vi "Set Input Volume.vi"(7 "Volume Mode (dB)":T1, 8 "error in (no error)":errorcluster, 9 "Volume":dbl, 10 "Input Name":string, 11 "OBS in":refnum<class "OBS.lvclass">) -> (0 "error out":errorcluster, 3 "OBS out":refnum<class "OBS.lvclass">)   [LabVIEW 2020, in "obs-websocket.lvlib" / "OBS.lvclass"]
uses:
  OBS.lvclass
  OBS.lvclass/OBS.ctl
  SetInputVolume/SetInputVolume.lvclass
  Volume Mode.ctl
  obs-websocket.lvlib
  C:/dev/lv20CE/lv-obs-websocket/obs-websocket-lv/Request/Request.lvclass
  C:/dev/lv20CE/lv-obs-websocket/obs-websocket-lv/Client Message/Client Message.lvclass
  C:/dev/lv20CE/lv-obs-websocket/obs-websocket-lv/Message/Message.lvclass
  C:/dev/lv20CE/lv-obs-websocket/obs-websocket-lv/SetInputVolume/SetInputVolume.lvclass
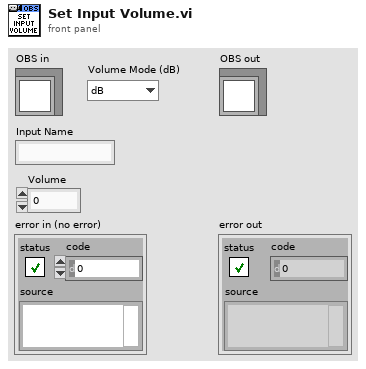
[diagram p1: front panel]
types:
  T1 = typedef "obs-websocket.lvlib/Volume Mode.ctl" = enum16{"dB", "Mul"}
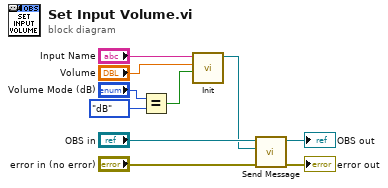
[diagram p0: block diagram]
diagram:
  n1 = Equal?(x="Volume Mode (dB)", y=Volume_Mode."dB") -> (x = y?=w1:bool)
  n2 = call "Init.vi"("Mode (F=Mul / T = dB)"=w1, "Volume"="Volume", "Input Name"="Input Name") -> ("SetInputVolume out"=w6:refnum<class "SetInputVolume.lvclass">)  [unwired: 7 in, 1 out]
  n3 = call "Send Message.vi"("error in (no error)"="error in (no error)", "Client Message"=w6, "OBS in"="OBS in") -> ("error out"=→"error out":errorcluster, "OBS in"=→"OBS out":refnum<class "OBS.lvclass">)  [unwired: 5 in, 2 out]
